vi "Last Cell.vi"(4 "Col Offset":i32, 6 "Row Offset":i32, 8 "Column":i32=-1, 9 "Row":i32=-1, 11 "Excel Sheet in":refnum<class "Excel Sheet.lvclass">) -> (0 "Column out":i32=-1, 1 "Row out":i32=-1, 2 "Cell":refnum<k7>, 3 "Excel Sheet out":refnum<class "Excel Sheet.lvclass">)   [LabVIEW 2016, in "Excel Sheet.lvclass"]
uses:
  Excel Sheet.lvclass
  Excel Sheet.lvclass/Excel Sheet.ctl
panel:
  out "error out":errorcluster
  in  "error in (no error)":errorcluster
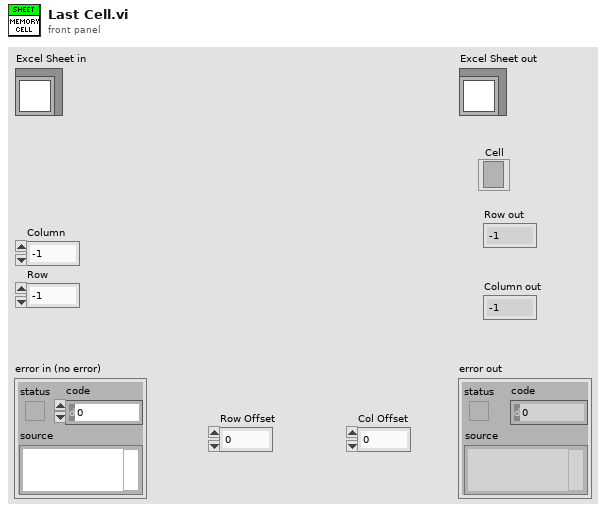
[diagram p1: front panel]
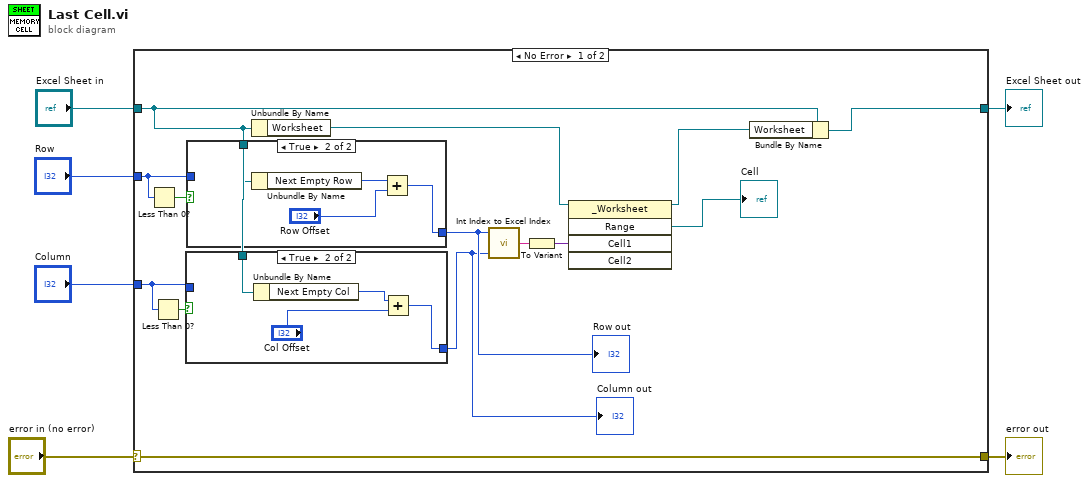
[diagram p0: block diagram]
diagram:
  n1 = case shown="No Error" "error in (no error)" {
    selector: "error in (no error)" -> [w20 w32]
    tunnel: [w20 w32] -> w5
    tunnel: [w16 w31] -> w3
    tunnel: "Excel Sheet in" -> [w11 w31]
    tunnel: "Column" -> [w13 _]
    tunnel: "Row" -> [w14 _]
    frame No Error {
      n2 = Less Than 0?(x=w14) -> (x < 0?=w15:bool)
      n3 = Less Than 0?(x=w13) -> (x < 0?=w12:bool)
      n4 = case shown="True" w12 {
        tunnel: w11 -> [_ w25]
        tunnel: [w21 w23] -> w8
        tunnel: w13 -> [w21 _]
        frame False {
        }
        frame True {
          n5 = Unbundle By Name(w25) -> ("Next Empty Col"=w24:i32)
          n6 = Add(x=w24, y="Col Offset") -> (x+y=w23:i32)
        }
      }
      "Column out" <- w8
      n7 = case shown="True" w15 {
        tunnel: w11 -> [_ w30]
        tunnel: [w26 w27] -> w9
        tunnel: w14 -> [w26 _]
        frame False {
        }
        frame True {
          n8 = Unbundle By Name(w30) -> ("Next Empty Row"=w29:i32)
          n9 = Add(x=w29, y="Row Offset") -> (x+y=w27:i32)
        }
      }
      "Row out" <- w9
      n10 = Unbundle By Name(w11) -> ("Worksheet"=w17:refnum<k7>)
      n11 = call "Int Index to Excel Index.vi"("Column"=w8, "Row"=w9) -> ("Cell"=w18:string)  [unwired: 3 in]
      n12 = To Variant(anything=w18) -> (Variant=w19:variant)
      n13 = invoke class="_Worksheet" method="Range"(reference=w17, "Cell1"=w19) -> (reference out=w10:refnum<k7>, "Range"=→"Cell":refnum<k7>)  [unwired: 3 in, 3 out]
      n14 = Bundle By Name(cluster=w11, "Worksheet"=w10) -> (w16:refnum<class "Excel Sheet.lvclass">)
    }
    frame Error {
    }
  }
  "error out" <- w5
  "Excel Sheet out" <- w3
